vi "Fire Buzzer.vi"(8 "error in (no error)":errorcluster) -> ()   [LabVIEW 2020]
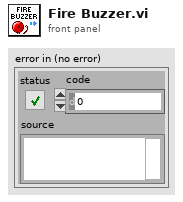
[diagram p1: front panel]
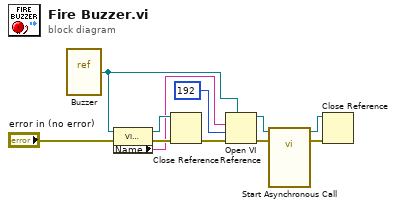
[diagram p0: block diagram]
diagram:
  n1 = vi-ref "Buzzer.vi"() -> (w5:refnum<vi>)
  n2 = property class="VI (strict)"(reference=w5, error in="error in (no error)") -> (reference out=w11:refnum<vi>, error out=w10:errorcluster, "Name"=w9:string)
  n3 = Close Reference(reference=w11, error in (no error)=w10) -> (error out=w3:errorcluster)
  n4 = Open VI Reference(type specifier VI Refnum (for type only)=w5, vi path=w9, options=192, error in (no error)=w3) -> (vi reference=w1:refnum<vi>, error out=w2:errorcluster)  [unwired: 2 in]
  n5 = call-by-ref "Start Asynchronous Call"(reference=w1, error in=w2) -> (reference out=w8:refnum<vi>, error out=w7:errorcluster)  [unwired: 12 in]
  n6 = Close Reference(reference=w8, error in (no error)=w7) -> ()  [unwired: 1 out]
